vi "Pre Launch Init.vi"(11 "DATABASE_MANEJO in":refnum<class "DATABASE_MANEJO.lvclass">) -> (0 "error out":errorcluster, 3 "DATABASE_MANEJO out":refnum<class "DATABASE_MANEJO.lvclass">)   [LabVIEW 2019, in "DATABASE_MANEJO.lvlib" / "DATABASE_MANEJO.lvclass"]
doc: "(<B>Filename</B>: Actor Framework.lvlib:Actor.lvclass:Pre Launch Init.vi)\n\nDefines behavior that occurs after the Launch Nested Actor method is invoked but before the actor's Actor Core method begins running.\n\nBy default, this method does nothing. A descendant class may override it to define behavior."
uses:
  DATABASE_MANEJO.lvclass
  DATABASE_MANEJO.lvclass/DATABASE_MANEJO.ctl
  <vilib>/ActorFramework/Actor/Actor.lvclass
panel:
  in  "Exit":bool
  in  "BASE DE DATOS":string
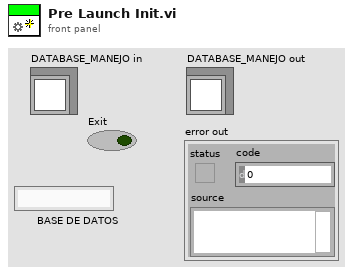
[diagram p1: front panel]
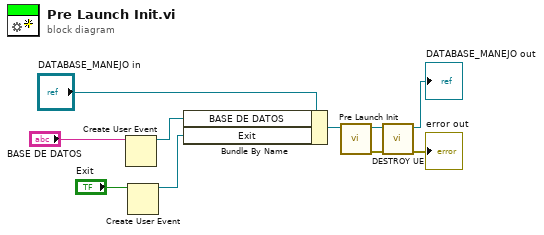
[diagram p0: block diagram]
diagram:
  n1 = Create User Event(user event datatype="BASE DE DATOS") -> (user event=w6:refnum<user-event>)  [unwired: 1 in, 1 out]
  n2 = Create User Event(user event datatype="Exit") -> (user event=w5:refnum<user-event>)  [unwired: 1 in, 1 out]
  n3 = Bundle By Name(cluster="DATABASE_MANEJO in", "BASE DE DATOS"=w6, "Exit"=w5) -> (w7:refnum<class "DATABASE_MANEJO.lvclass">)
  n4 = call-parent "Pre Launch Init.vi"("Actor in"=w7) -> ("error out"=w4:errorcluster, "Actor out"=w2:refnum<class "DATABASE_MANEJO.lvclass">)  [unwired: 9 in]
  n5 = call "DESTROY UE.vi"("error in (no error)"=w4, "DATABASE_MANEJO in"=w2) -> ("error out"=→"error out":errorcluster, "DATABASE_MANEJO out"=→"DATABASE_MANEJO out":refnum<class "DATABASE_MANEJO.lvclass">)  [unwired: 8 in]
